vi "CMN_toDSENDER.vi"(4 "nelems":u32, 6 "data":string, 7 "pointer":u64, 8 "error in (no error)":errorcluster, 9 "ms timeout (-1)":i32=-1, 10 "responseQ":string, 11 "Command":string) -> (0 "error out":errorcluster, 2 "response":string)   [LabVIEW 2016]
panel:
  in  "cmdstruct":T1
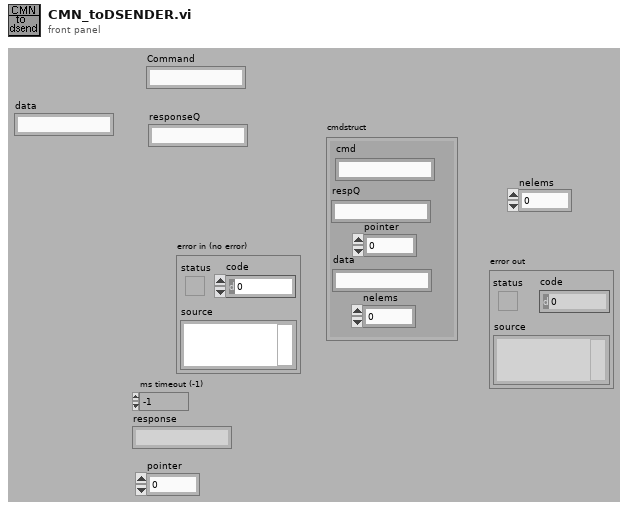
[diagram p1: front panel]
types:
  T1 = cluster{"cmd":string, "respQ":string, "pointer":u64, "data":string, "nelems":u32}
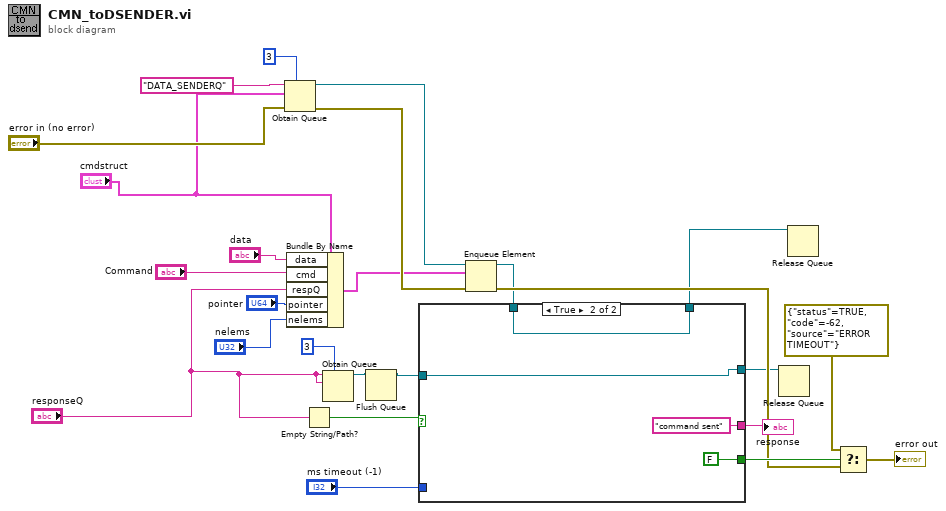
[diagram p0: block diagram]
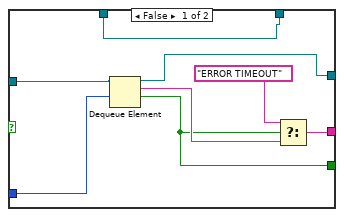
[diagram p2: hidden frame]
diagram:
  n1 = Obtain Queue(max queue size (-1, unlimited)=3, name (unnamed)="DATA_SENDERQ", element data type="cmdstruct", error in (no error)="error in (no error)") -> (queue out=w24:refnum<queue>, error out=w18:errorcluster)  [unwired: 1 in, 1 out]
  n2 = Bundle By Name(cluster="cmdstruct", "data"="data", "cmd"="Command", "respQ"="responseQ", "pointer"="pointer", "nelems"="nelems") -> (w10:T1)
  n3 = Empty String/Path?(string/path="responseQ") -> (empty?=w22:bool)
  n4 = Obtain Queue(max queue size (-1, unlimited)=3, name (unnamed)="responseQ", element data type="responseQ") -> (queue out=w6:refnum<queue>)  [unwired: 2 in, 2 out]
  n5 = Flush Queue(queue=w6) -> (queue out=w4:refnum<queue>)  [unwired: 1 in, 2 out]
  n6 = Enqueue Element(queue=w24, element=w10, error in (no error)=w18) -> (queue out=w7:refnum<queue>, error out=w14:errorcluster)  [unwired: 2 out]
  n7 = case shown="True" w22 {
    tunnel: "ms timeout (-1)" -> [w33 _]
    tunnel: [w30 "command sent"] -> w20
    tunnel: [w29 FALSE ("timed out?")] -> w17
    tunnel: [w28 w35] -> w8
    tunnel: w7 -> [w28 w35]
    tunnel: w4 -> [w27 w34]
    tunnel: [w26 w34] -> w3
    frame False {
      n8 = Dequeue Element(queue=w27, timeout in ms (-1)=w33) -> (queue out=w26:refnum<queue>, element=w32:string, timed out?=w29:bool)  [unwired: 1 in, 1 out]
      n9 = Select(t="ERROR TIMEOUT", s=w29, f=w32) -> (s? t:f=w30:string)
    }
    frame True {
    }
  }
  "response" <- w20
  n10 = Release Queue(queue=w3) -> ()  [unwired: 1 in, 4 out]
  n11 = Release Queue(queue=w8) -> ()  [unwired: 1 in, 4 out]
  n12 = Select(t=errorcluster {"status"=TRUE, "code"=-62, "source"="ERROR TIMEOUT"}, s=w17, f=w14) -> (s? t:f=→"error out":errorcluster)
